vi "GetJSON.vi"(8 "Error In":errorcluster, 10 "Controls?":bool, 11 "VI Refnum In":refnum<vi>) -> (0 "Error Out":errorcluster, 2 "JSON Out":string, 3 "VI Refnum Out":refnum<vi>)   [LabVIEW 2019, in "LabJSON.lvlib"]
doc: "Get JSON of all controls/indicators for a given VI."
uses:
  LabJSON.lvlib
  <vilib>/JDP Science/JSONtext/JSONtext.lvlib
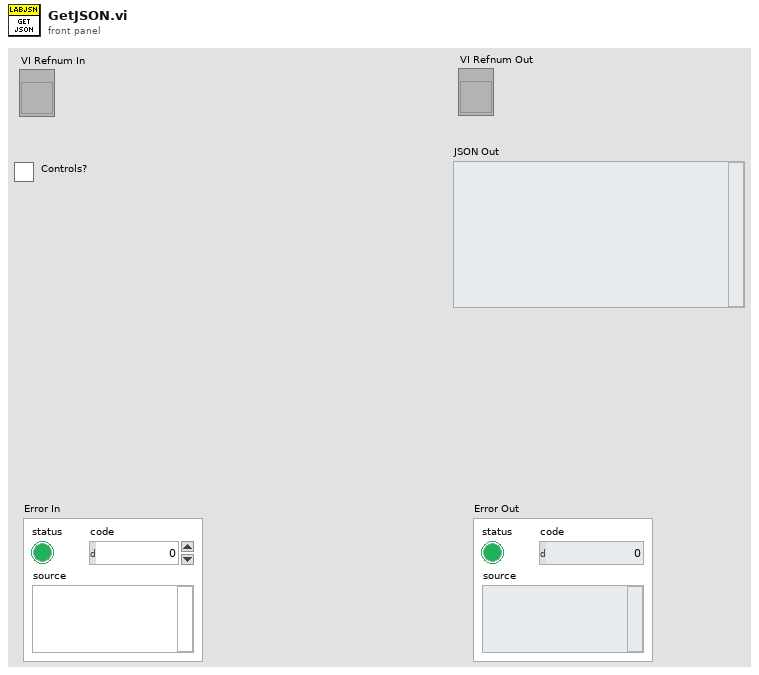
[diagram p1: front panel]
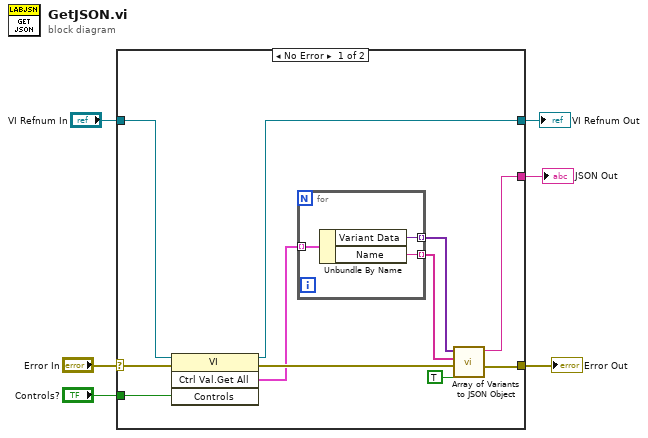
[diagram p0: block diagram]
diagram:
  n1 = case shown="No Error" "Error In" {
    selector: "Error In" -> [w12 w22]
    tunnel: [w8 w22] -> w5
    tunnel: "VI Refnum In" -> [w11 w21]
    tunnel: [w10 _] -> w3
    tunnel: [w9 w21] -> w2
    tunnel: "Controls?" -> [w7 _]
    frame No Error {
      n2 = invoke class="VI" method="Ctrl Val.Get All"(reference=w11, error in=w12, "Controls"=w7) -> (reference out=w9:refnum<vi>, error out=w17:errorcluster, "Get All Control Values Variant"=w14:cluster{"Name":string, "Variant Data":variant}[])  [unwired: 1 in, 1 out]
      n3 = for {
        tunnel: w14 -> [w20] mode=indexing
        tunnel: [w19] -> w16 mode=indexing
        tunnel: [w18] -> w15 mode=indexing
        n4 = Unbundle By Name(w20) -> ("Variant Data"=w19:variant, "Name"=w18:string)
      }
      n5 = call <vilib>:"Array of Variants to JSON Object.vi"("Pretty Print?"=TRUE, "error in (no error)"=w17, "Names"=w15, "Array"=w16) -> ("error out"=w8:errorcluster, "<JSON>"=w10:string)  [unwired: 6 in]
    }
    frame Error {
    }
  }
  "JSON Out" <- w3
  "Error Out" <- w5
  "VI Refnum Out" <- w2
